vi "DataFinder_DisplaySensorResults.vi"(1 "result references":T2[](array[typedef]), 2 "results elements":T1, 3 "error in":errorcluster) -> ()   [LabVIEW 2023]
doc: "Displays search results of query for Sensor_Type."
uses:
  <vilib>/userdefined/DFSearchResult.ctl
  <vilib>/DataFinder/DataTypes/results elements.ctl
  <vilib>/DataFinder/DataTypes/object type.ctl
  <vilib>/DataFinder/DataTypes/property.ctl
  <vilib>/DataFinder/DataTypes/data type.ctl
  <vilib>/Utility/error.llb/DialogType.ctl
  <vilib>/DataFinder/Get Property Values (String Property).vi
  <vilib>/DataFinder/Close Reference (Results).vi
  <vilib>/DataFinder/NI_DataFinder.lvlib
  <vilib>/userdefined/NI_DataFinder Controls.lvlib
panel:
  out "error text":string=" INSTRUCTIONS:\r\rNormal Use:  When using subVIs that incorporate the error in/error out (or error I/O) structure, place this handler where you want to inform the user of an error, typically at the end of the I/O data path, as the last action of the program.  If the error in error? is ERROR, the handler creates a message describing the error and its source.  If the type of dialog = 1 (default), the message is displayed to the user, who can only acknowedge it.  If the type = 2, the user can acknowledge the message or abort execution; aborting a program with active I/O is not recommended.  If the type = 0, no message is displayed; this is used to process the error programmatically, and the error out cluster elements are wired to individual terminals for that reason.  \r\rOther Use:\n\r\nlocal testing.  To test the error code of a subVI or function that does not have the error I/O structure, you can wire its error code and a source string to the local error code and error source inputs.  If error in error? indicates no error and error code is not equal to 0, the local code and source are substituted for the error in values, and error? is set TRUE (ERROR)."
  in  "Close":bool
  in  "Table Control":string[][](table) caption="Search Results"
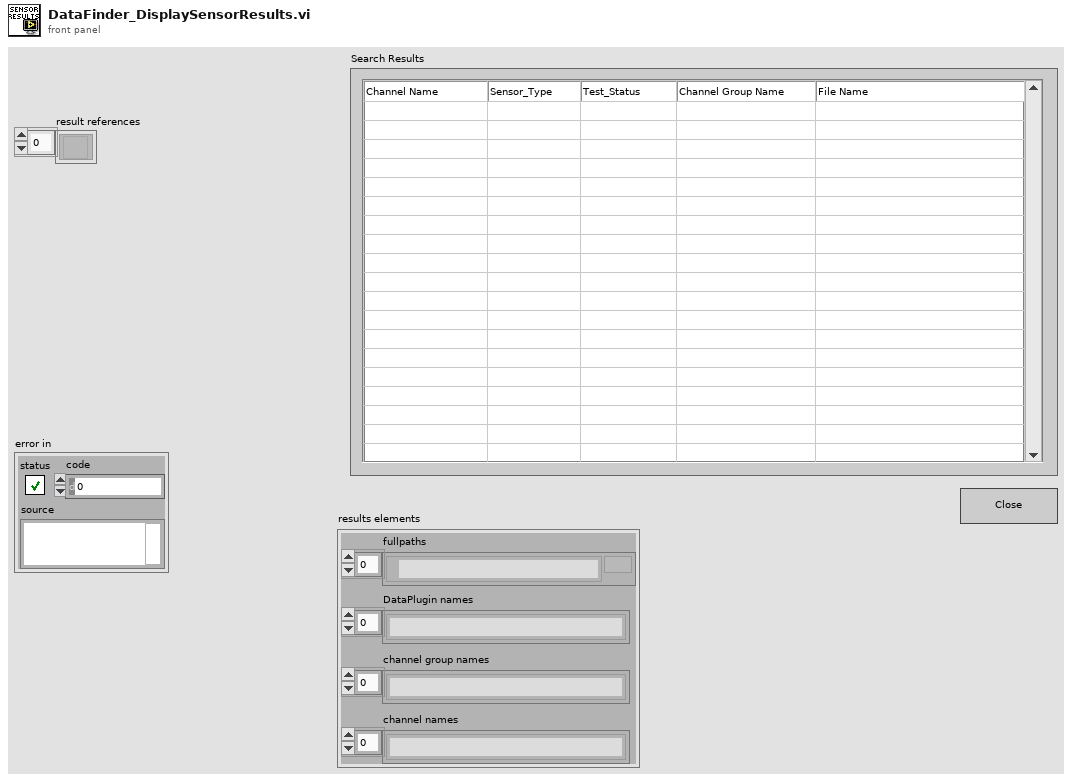
[diagram p1: front panel]
types:
  T1 = typedef "NI_DataFinder.lvlib/results elements.ctl" = cluster{"fullpaths":path[], "DataPlugin names":string[], "channel group names":string[], "channel names":string[]}
  T2 = typedef "NI_DataFinder Controls.lvlib/DFSearchResult.ctl" = refnum<k20>
  T3 = typedef "NI_DataFinder.lvlib/property.ctl" = cluster{"object type":T4, "property name":string, "data type":T5}
  T4 = typedef "NI_DataFinder.lvlib/object type.ctl" = u16
  T5 = typedef "NI_DataFinder.lvlib/data type.ctl" = u16
  T6 = typedef "DialogType.ctl" = u16
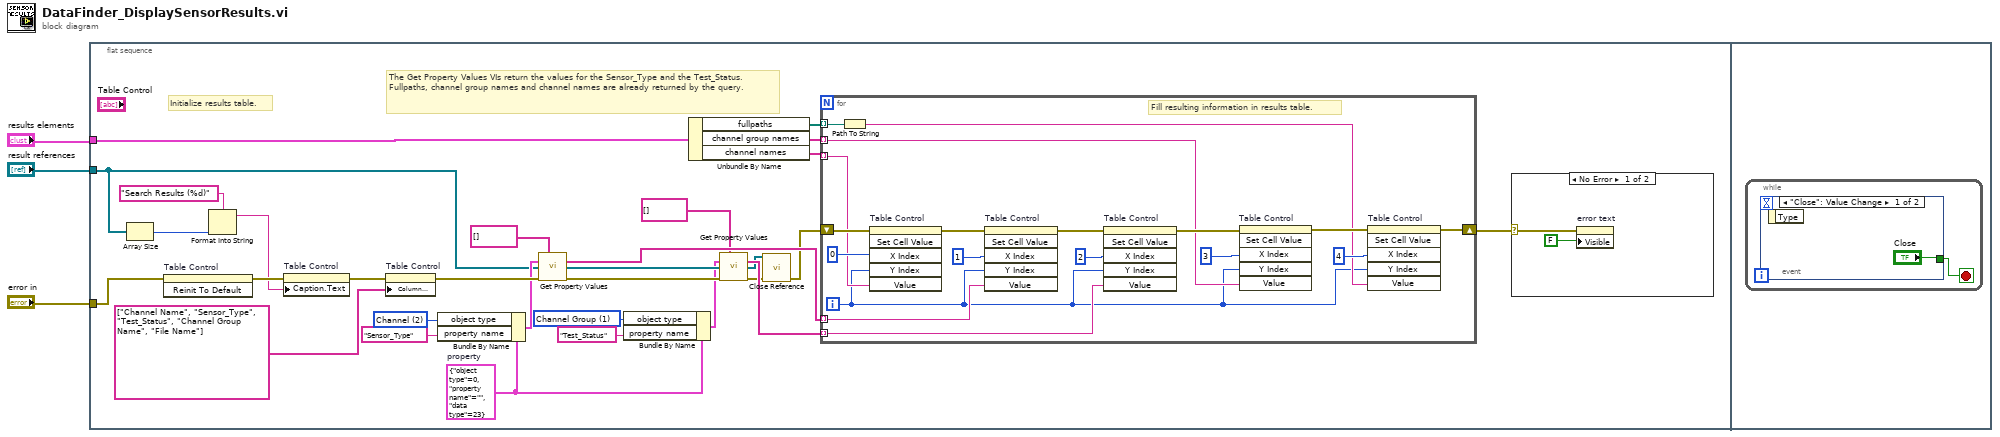
[diagram p0: block diagram]
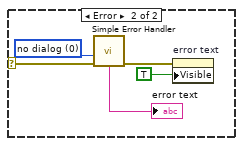
[diagram p2: hidden frame]
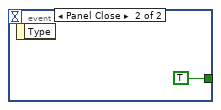
[diagram p3: hidden frame]
diagram:
  n1 = flat-sequence {
    tunnel: "results elements" -> [w13]
    tunnel: "result references" -> [w12]
    tunnel: "error in" -> [w11]
    frame #0 {
      w4 = T3 {"object type"=0, "property name"="", "data type"=23}  # property
      w15 = T4 1 items=["File", "Channel Group", "Channel"] ("object type")
      w19 = T4 2 items=["File", "Channel Group", "Channel"] ("object type")
      # "Initialize results table."
      # "The Get Property Values VIs return the values for the Sensor_Type and the Test_Status. Fullpaths, channel group names and channel names are already returned by the query."
      n2 = Array Size(array=w12) -> (size(s)=w7:i32)
      n3 = invoke on="Table Control" class="Tbl (strict)" method="Reinit To Default"(error in=w11) -> (error out=w24:errorcluster)  [unwired: 2 in, 2 out]
      n4 = Format Into String(format string="Search Results (%d)" ("string"), w7) -> (resulting string=w6:string)  [unwired: 2 in, 1 out]
      n5 = property on="Table Control" class="Tbl (strict)"(error in=w24, "Caption.Text"=w6) -> (error out=w22:errorcluster)  [unwired: 1 in, 1 out]
      n6 = property on="Table Control" class="Tbl (strict)"(error in=w22, "Column Headers[]"=string[] ["Channel Name", "Sensor_Type", "Test_Status", "Channel Group Name", "File Name"] ("Column Header Strings[]")) -> (error out=w20:errorcluster)  [unwired: 1 in, 1 out]
      n7 = Bundle By Name(cluster=w4, "object type"=w19, "property name"="Sensor_Type") -> (w18:T3)
      n8 = call-poly <vilib>:"Get Property Values.vi"("data type"=string[] [], "property"=w18, "result references"=w12, "error in (no error)"=w20) -> ("property values"=w27:string[], "result references out"=w30:T2[], "error out"=w29:errorcluster)  [unwired: 9 in]
      n9 = Bundle By Name(cluster=w4, "object type"=w15, "property name"="Test_Status") -> (w16:T3)
      n10 = Unbundle By Name(w13) -> ("fullpaths"=w31:path[], "channel group names"=w32:string[], "channel names"=w33:string[])
      n11 = call-poly <vilib>:"Get Property Values.vi"("data type"=string[] [], "property"=w16, "result references"=w30, "error in (no error)"=w29) -> ("property values"=w26:string[], "result references out"=w8:T2[], "error out"=w10:errorcluster)  [unwired: 9 in]
      n12 = call-poly <vilib>:"Close Reference.vi"("result references"=w8, "error in (no error)"=w10) -> ("error out"=w9:errorcluster)  [unwired: 13 in]
      n13 = for {
        tunnel: w33 -> [w47] mode=indexing
        shift-right: [w41] -> w23
        shift-left: w9 -> [w57]
        tunnel: w32 -> [w44] mode=indexing
        tunnel: w31 -> [w48] mode=indexing
        tunnel: w27 -> [w46] mode=indexing
        tunnel: w26 -> [w45] mode=indexing
        i -> [w42]
        # "Fill resulting information in results table."
        n14 = Path To String(path=w48) -> (string=w43:string)
        n15 = invoke on="Table Control" class="Tbl (strict)" method="Set Cell Value"(error in=w57, "X Index"=u32 0, "Y Index"=w42, "Value"=w47) -> (error out=w53:errorcluster)  [unwired: 2 in, 5 out]
        n16 = invoke on="Table Control" class="Tbl (strict)" method="Set Cell Value"(error in=w53, "X Index"=u32 1, "Y Index"=w42, "Value"=w46) -> (error out=w52:errorcluster)  [unwired: 2 in, 5 out]
        n17 = invoke on="Table Control" class="Tbl (strict)" method="Set Cell Value"(error in=w52, "X Index"=u32 2, "Y Index"=w42, "Value"=w45) -> (error out=w51:errorcluster)  [unwired: 2 in, 5 out]
        n18 = invoke on="Table Control" class="Tbl (strict)" method="Set Cell Value"(error in=w51, "X Index"=u32 3, "Y Index"=w42, "Value"=w44) -> (error out=w50:errorcluster)  [unwired: 2 in, 5 out]
        n19 = invoke on="Table Control" class="Tbl (strict)" method="Set Cell Value"(error in=w50, "X Index"=u32 4, "Y Index"=w42, "Value"=w43) -> (error out=w41:errorcluster)  [unwired: 2 in, 5 out]
      }
      n20 = case shown="No Error" w23 {
        selector: w23 -> [w35 w40]
        frame No Error {
          n21 = property on="error text" class="Str"(error in=w35, "Visible"=FALSE) -> ()  [unwired: 1 in, 2 out]
        }
        frame Error {
          w39 = T6 0 items=["no dialog", "OK message", "continue or stop message", "OK message + warnings", "continue/stop + warnings"] ("type of dialog (OK msg:1)")
          n22 = call <vilib>:"Simple Error Handler.vi"("type of dialog (OK msg:1)"=w39, "error in (no error)"=w40) -> ("error out"=w36:errorcluster, "message"=→"error text":string)  [unwired: 6 out]
          n23 = property on="error text" class="Str"(error in=w36, "Visible"=TRUE) -> ()  [unwired: 1 in, 2 out]
        }
      }
    }
    frame #1 {
      n24 = while {
        stop <- w59 stop-if-true
        n25 = event shown="[0] \"Close\": Value Change" {
          selector: _ -> [_ _]
          dyn-events: _ -> [_ _]
          timeout: _ -> [_ _]
          tunnel: ["Close" TRUE ("Cancel")] -> w59
          event "Close": Value Change {
            n26 = event-data() -> ()  [unwired: 2 out]
          }
          event Panel Close {
            n27 = event-data() -> ()  [unwired: 2 out]
          }
        }
      }
    }
  }
